vi "PS-OCTA-OCE-autofocus.vi"() -> ()   [LabVIEW 2024] (continued)
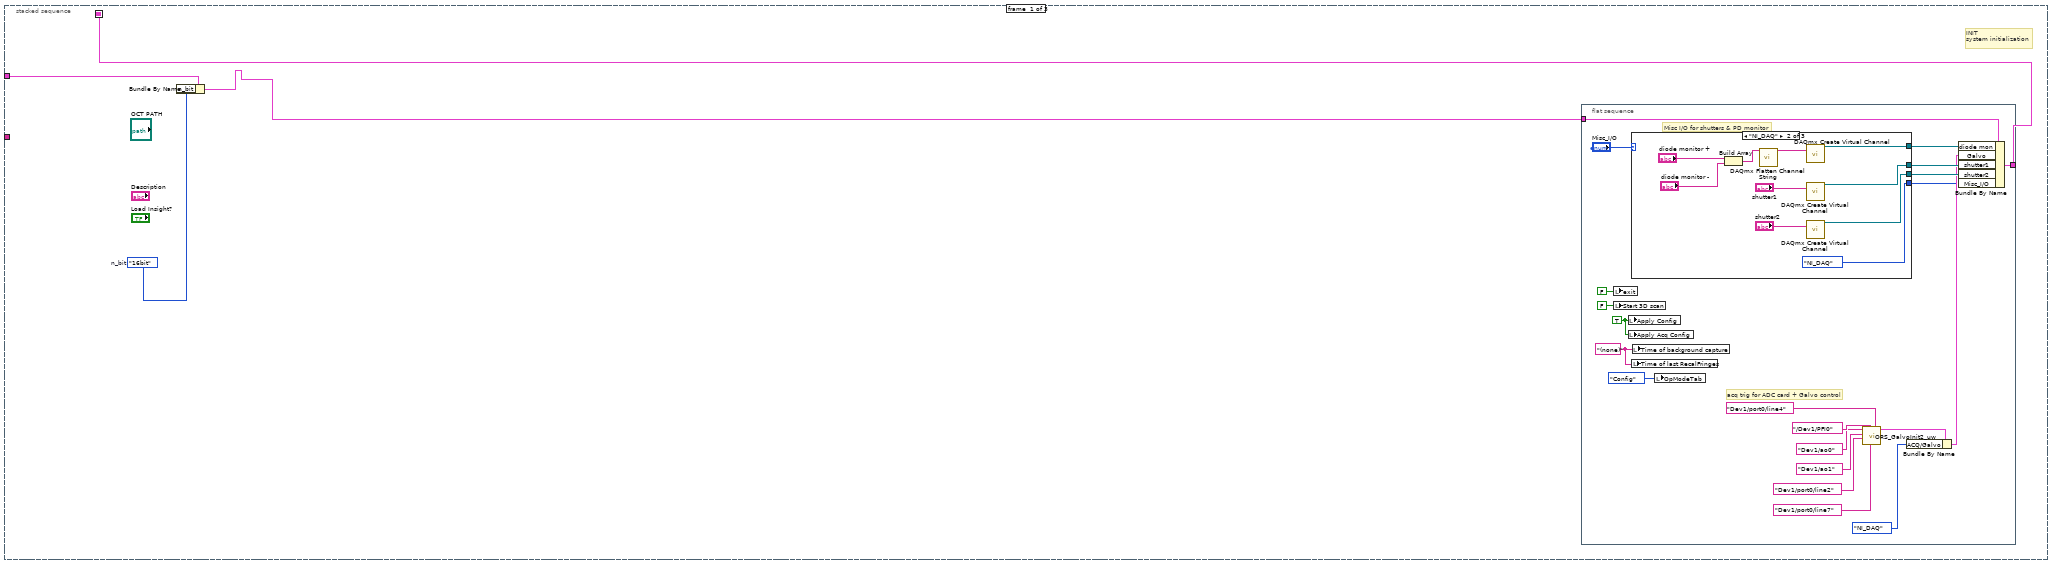
[diagram p3: hidden frame]
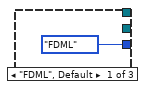
[diagram p4: hidden frame]
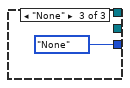
[diagram p5: hidden frame]
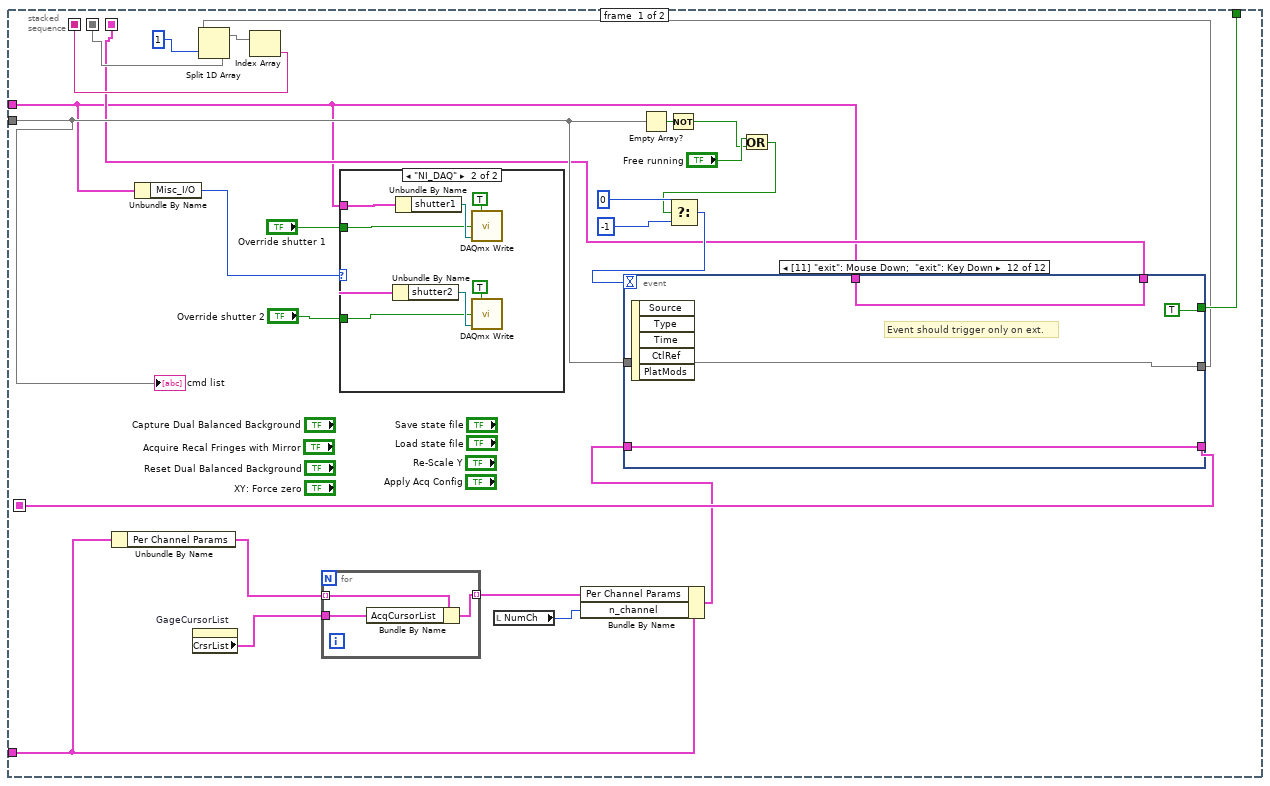
[diagram p7: hidden frame]
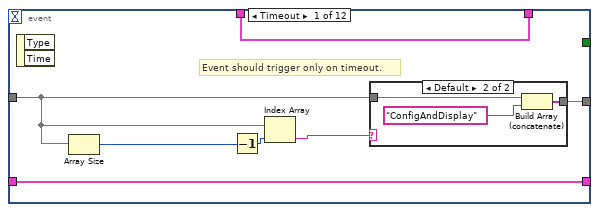
[diagram p9: hidden frame]
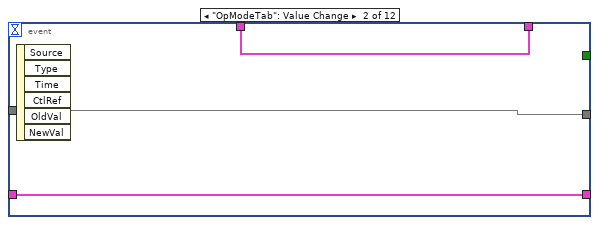
[diagram p11: hidden frame]
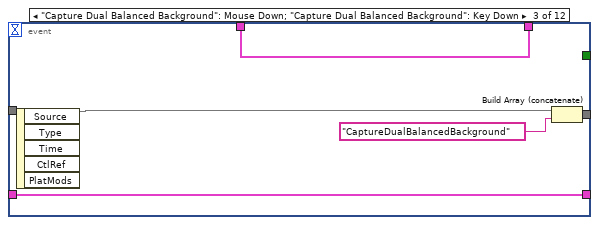
[diagram p12: hidden frame]
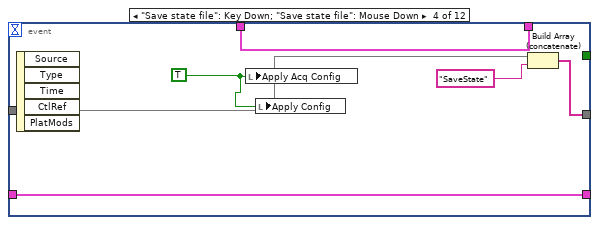
[diagram p13: hidden frame]
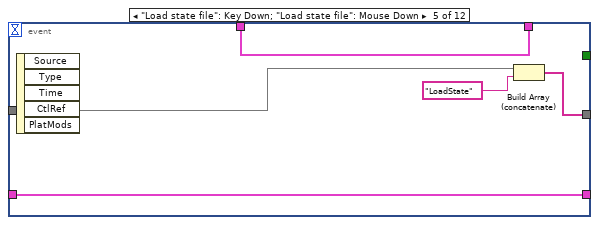
[diagram p14: hidden frame]
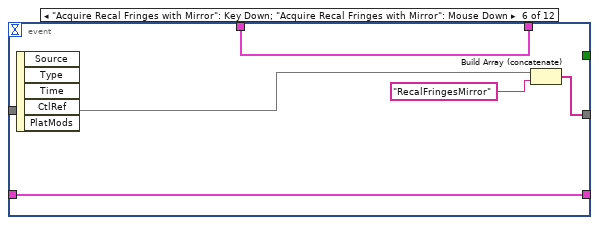
[diagram p15: hidden frame]
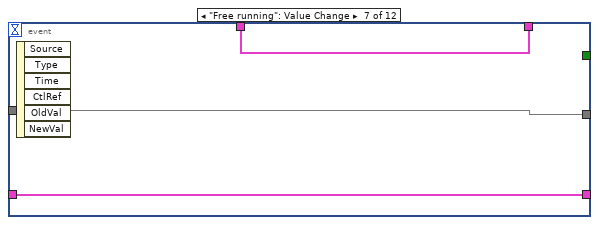
[diagram p16: hidden frame]
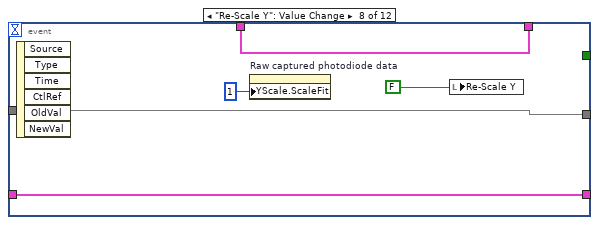
[diagram p17: hidden frame]
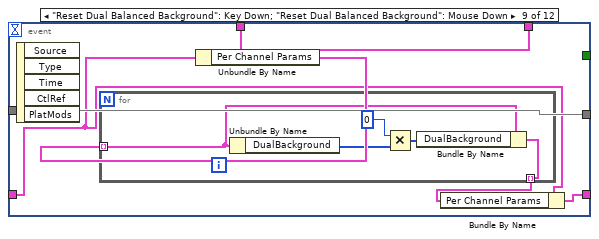
[diagram p18: hidden frame]
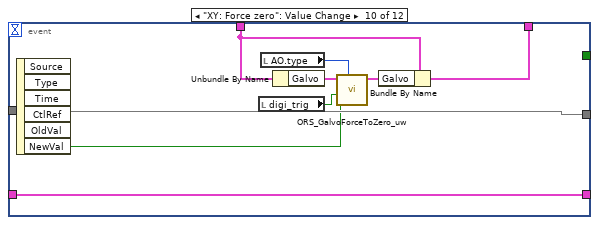
[diagram p19: hidden frame]
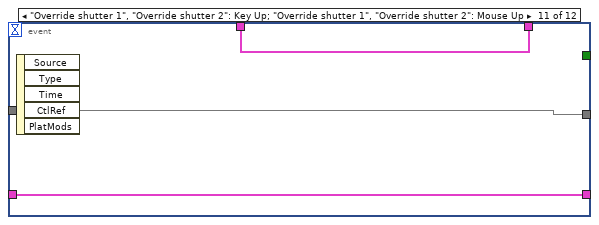
[diagram p20: hidden frame]
                    # "data transfer end timer"
                    # "acq start timer"
                    # "#AllocatedBuffer"
                    n725 = stacked-sequence {
                      seq-local: [_ w1514 _ _ _] -> [_ _ w1706 _ _]
                      seq-local: [_ w1520 _ _ _] -> [_ _ w1703 _ w1985]
                      seq-local: [_ w1519 _ _ _] -> [_ _ w1702 _ _]
                      seq-local: [_ w1518 _ _ _] -> [_ _ _ w1961 _]
                      seq-local: [_ _ w1701 _ _] -> [_ _ _ w1960 _]
                      seq-local: [_ _ w1700 _ _] -> [_ _ _ w1955 _]
                      seq-local: [_ _ w1699 _ _] -> [_ _ _ w1953 _]
                      seq-local: [_ _ w1698 _ _] -> [_ _ _ w1957 _]
                      seq-local: [_ w1517 _ _ _] -> [_ _ w1697 _ _]
                      seq-local: [_ w1516 _ _ _] -> [_ _ _ w1950 _]
                      seq-local: [_ w1515 _ _ _] -> [_ _ w1691 _ _]
                      seq-local: [_ w1513 _ _ _] -> [_ _ w1696 _ _]
                      seq-local: [_ w1512 _ _ _] -> [_ _ w1695 _ _]
                      seq-local: [_ w1511 _ _ _] -> [_ _ w1694 _ _]
                      seq-local: [_ w1510 _ _ _] -> [_ _ w1693 _ _]
                      seq-local: [_ w1509 _ _ _] -> [_ _ w1692 _ _]
                      seq-local: [w1499 _ _ _ _] -> [_ w1508 _ _ _]
                      seq-local: [_ w1507 _ _ _] -> [_ _ w1690 _ _]
                      tunnel: w1496 -> [w1502 _ _ _ _]
                      tunnel: [_ _ _ _ w1987] -> w1495
                      tunnel: w1494 -> [_ w1521 w1707 _ w1975]
                      tunnel: [_ _ _ _ w1975] -> w1493
                      tunnel: w1492 -> [_ _ w1705 _ _]
                      tunnel: w1491 -> [_ _ w1704 _ _]
                      frame #0 {
                        n726 = local read "ATSHandle"() -> (w1497:u32[])
                        n727 = Unbundle By Name(w1502) -> ("Galvo"=w1500:T5)
                        n728 = call "ORS_GalvoCleanupScan.vi"("Galvo"=w1500) -> ("Galvo out"=w1501:T5)  [unwired: 9 in, 1 out]
                        n729 = for {
                          tunnel: [w1506] -> w1498
                          tunnel: w1497 -> [w1503] mode=indexing
                          n730 = call "AlazarAbortCapture.vi"("Handle"=w1503) -> ("Handle"=w1505:u32, "error out"=w1504:errorcluster)  [unwired: 1 in, 1 out]
                          n731 = call "AlazarAbortAsyncRead.vi"("Handle"=w1505, "error in (no error)"=w1504) -> ("error out"=w1506:errorcluster)  [unwired: 2 out]
                        }
                        n732 = Bundle By Name(cluster=w1502, "Galvo"=w1501) -> (w1499:T6)
                        n733 = call <vilib>:"Simple Error Handler.vi"("error in (no error)"=w1498) -> ()  [unwired: 4 in, 5 out]
                      }
                      frame #1 {
                        n734 = stacked-sequence {
                          seq-local: [w1556 _ _ _ _] -> [_ w1625 _ _ _]
                          seq-local: [w1548 _ _ _ _] -> [_ w1629 _ _ _]
                          seq-local: [w1547 _ _ _ _] -> [_ w1628 _ _ _]
                          seq-local: [w1546 _ _ _ _] -> [_ w1627 _ _ _]
                          seq-local: [w1542 _ _ _ _] -> [_ w1626 _ _ _]
                          seq-local: [w1541 _ _ _ _] -> [_ w1588 _ _ _]
                          seq-local: ["3D frame" _ _ _ _] -> [_ w1608 _ _ _]
                          seq-local: ["B_frames per trigger" _ _ _ _] -> [_ w1607 _ _ _]
                          seq-local: [_ w1629 _ _ _] -> [_ _ w1676 _ _]
                          seq-local: [_ w1625 _ _ _] -> [_ _ w1675 _ _]
                          seq-local: [_ w1628 _ _ _] -> [_ _ w1674 _ _]
                          seq-local: [_ w1627 _ _ _] -> [_ _ w1673 _ _]
                          seq-local: [_ _ w1675 _ _] -> [_ _ _ w1684 _]
                          seq-local: [_ _ _ w1684 _] -> [_ _ _ _ w1687]
                          tunnel: w1508 -> [w1557 _ _ _ _]
                          tunnel: w1521 -> [w1541 _ _ _ _]
                          tunnel: [w1548 _ _ _ _] -> w1519
                          tunnel: [w1545 _ _ _ _] -> w1517
                          tunnel: [w1535 _ _ _ _] -> w1515
                          tunnel: [w1543 _ _ _ _] -> w1514
                          tunnel: [w1539 _ _ _ _] -> w1507
                          tunnel: [_ w1610 _ _ _] -> w1513
                          tunnel: [_ w1612 _ _ _] -> w1512
                          tunnel: [_ w1624 _ _ _] -> w1511
                          tunnel: [_ w1623 _ _ _] -> w1510
                          tunnel: [_ w1616 _ _ _] -> w1509
                          tunnel: [_ _ w1672 _ _] -> w1516
                          tunnel: [_ _ _ _ w1686] -> w1520
                          tunnel: [_ _ _ _ w1685] -> w1518
                          frame #0 {
                            (unwired) u32 0 ("y")
                            w1538 = 10178 items=["Finite Samples"=10178, "Continuous Samples"=10123, "Hardware Timed Single Point"=12522] ("SampQuant.SampMode")
                            # "Trigger condition: 0 =  transducer ON for the scan"
                            n735 = case shown="False" "3D: dummy/real" {
                              tunnel: [w1560 w1561] -> w1548
                              tunnel: T12."Alazar" ("Data source") -> [w1558 w1561]
                              frame False {
                                n736 = Type Cast(type=w1558, x=9999) -> (*(type *) &x=w1560:T12)
                              }
                              frame True {
                              }
                            }
                            n737 = Unbundle By Name(w1557) -> ("Galvo"=w1552:T5)
                            n738 = local read "3D_Galvo_Params"() -> (w1527:T4)
                            n739 = local read "XY: Force zero"() -> (w1551:bool)
                            n740 = Bundle By Name(cluster=w1552, "params"=w1527, "params.force to zero"=w1551, "params.Triggers_per_sweep"=1.0) -> (w1550:T5)
                            n741 = Unbundle By Name(w1527) -> ("mode"=w1525:i32)
                            n742 = Subtract(x=w1525, y=7) -> (x-y=w1523:i32)
                            n743 = Multiply(x=w1523, y=-1) -> (x*y=w1522:i32)
                            n744 = local read "digi_trig"() -> (w1537:bool)
                            n745 = call "ORS_GalvoConfig3D_v2.vi"("Galvo"=w1550, "use_digi_trig"=w1537) -> ("Galvo out"=w1531:T5, "error out"=w1554:errorcluster)  [unwired: 16 in]
                            n746 = local read "Slow axis-----Fast axis"() -> (w1528:bool)
                            n747 = local read "AO.type"() -> (w1533:i32)
                            n748 = call "ORS_GalvoPrepareScan_uw-1kp_Duo.vi"("Galvo"=w1531, "SampQuant.SampMode"=w1538, "3D frame"="3D frame", "AO.DataXferMech"=w1533, "Fast Axis/Slow Axis"=w1528, "use_digi_trig"=w1537, "error in"=w1554, "Trigger condition"=w1522) -> ("Galvo out"=w1532:T5, "error out"=→"error out":errorcluster)  [unwired: 4 in, 2 out]
                            n749 = Unbundle By Name(w1532) -> ("params.n_lines"=w1553:i32, "params.n_frames"=w1536:i32)
                            n750 = Bundle By Name(cluster=w1557, "Galvo"=w1532) -> (w1556:T6)
                            n751 = case shown="\"Alazar\"" w1548 {
                              tunnel: w1536 -> [_ w1576]
                              tunnel: w1553 -> [_ w1579]
                              tunnel: [-1.0 w1573] -> w1542
                              tunnel: [_ w1565] -> w1547
                              tunnel: [_ w1578] -> w1546
                              tunnel: [_ w1575] -> w1545
                              tunnel: [_ w1574] -> w1543
                              tunnel: [_ w1567] -> w1539
                              tunnel: [_ w1566] -> w1534
                              frame Default {
                              }
                              frame "Alazar" {
                                n752 = Multiply(x=w1576, y=w1579) -> (x*y=w1571:i32)
                                n753 = Multiply(x=w1571, y=1) -> (x*y=w1570:i32)
                                n754 = local read "Laser Trigger"() -> (w1563:bool)
                                n755 = local read "ATSHandle"() -> (w1565:u32[])
                                n756 = local read "# samples"() -> (w1573:u32)
                                n757 = local read "Channel"() -> (w1572:u32)
                                n758 = for {
                                tunnel: w1565 -> [w1587] mode=indexing
                                tunnel: w1579 -> [w1586]
                                tunnel: [w1585] -> w1578
                                tunnel: w1573 -> [w1584]
                                tunnel: w1572 -> [w1583]
                                tunnel: w1570 -> [w1582]
                                tunnel: [w1581] -> w1564
                                tunnel: w1563 -> [w1580]
                                n759 = call "ORS_AlazarDLLAcq_Prepare.vi"("Lamda Trigger?"=w1580, "Channel"=w1583, "Records Per Buffer"=w1586, "Records Count"=w1582, "Record length"=w1584, "ATSHandle"=w1587) -> ("error out"=w1585:errorcluster, "Samps Per Buffer"=w1581:u32)  [unwired: 3 in, 1 out]
                                }
                                n760 = Array Size(array=w1565) -> (size(s)=w1566:i32)
                                n761 = Multiply(x=w1564, y=w1566) -> ()  [unwired: 1 out]
                                n762 = Initialize Array(i16 0 ("element"), w1564) -> (w1575:i16[])
                                n763 = Obtain Queue(element data type=w1575) -> (queue out=w1574:refnum<queue>)  [unwired: 4 in, 2 out]
                                n764 = Multiply(x=w1564, y=u32 2) -> (x*y=w1567:u32)
                              }
                            }
                            "samples/line 3d" <- w1542
                            n765 = Multiply(x=w1536, y=w1534) -> (x*y=w1535:i32)
                          }
                          frame #1 {
                            # "File suffix to add angle, type of acquisition and extension to the file name"
                            n766 = local read "OCTA_indicator"() -> (w1595:bool)
                            n767 = local read "Current Angle"() -> (w1605:dbl)
                            n768 = call "ORS_timestamp.vi"() -> ("system time"=w1620:string)
                            n769 = call "ORS_DatafileWriteReadHeader_OCE.vi"() -> ("Parameter Cluster v8"=w1609:T27, "error out"=w1606:errorcluster)  [unwired: 17 in, 1 out]
                            n770 = stacked-sequence {
                              seq-local: [w1640 _] -> [_ w1650]
                              tunnel: w1609 -> [w1634 _]
                              tunnel: w1625 -> [w1642 _]
                              tunnel: w1626 -> [w1641 _]
                              tunnel: [_ w1653] -> w1613
                              tunnel: w1588 -> [w1638 w1652]
                              tunnel: [_ w1647] -> w1623
                              tunnel: [_ w1645] -> w1624
                              tunnel: [_ w1644] -> w1616
                              frame #0 {
                                n771 = Unbundle By Name(w1638) -> ("Sample Rate"=w1639:dbl)
                                n772 = local read "Description"() -> (w1630:string)
                                n773 = local read "file version"() -> (w1636:u32)
                                n774 = local read "image height"() -> (w1635:i32)
                                n775 = Unbundle By Name(w1642) -> ("Galvo"=w1633:T5)
                                n776 = local read "n_bit"() -> (w1632:enum16{"8bit", "16bit"})
                                n777 = Bundle By Name(cluster=w1634, "Galvo"=w1633, "description"=w1630, "samples_per_line"=w1641, "sampling_rate"=w1639, "vert_range"=0.0, "image height (crop)"=w1635, "file version"=w1636, "data set dimension"=u16 1, "n_bit"=w1632) -> (w1640:T27)
                              }
                              frame #1 {
                                n778 = Unbundle By Name(w1652) -> ("Per Channel Params"=w1649:T8)
                                n779 = Index Array(array=w1649) -> (element=w1643:T13)  [unwired: 1 in]
                                n780 = local read "DoInterp"() -> (w1646:bool)
                                n781 = local read "NumCh"() -> (w1651:i32)
                                n782 = Unbundle By Name(w1643) -> ("DualBackground"=w1644:i16[], "RecalFringePhaseFit"=w1648:dbl[][])
                                n783 = Bundle By Name(cluster=w1650, "n_channel"=w1651, "Per Channel Params"=w1649) -> (w1653:T27)
                                n784 = case shown="False" w1646 {
                                tunnel: w1648 -> [w1656 w1665]
                                tunnel: [w1655 w1663] -> w1647
                                tunnel: [w1654 w1663] -> w1645
                                frame True {
                                n785 = Index Array(array=w1656, index (row)=0) -> (element=w1654:dbl[])  [unwired: 1 in]
                                n786 = Array Size(array=w1654) -> (size(s)=w1660:i32)
                                n787 = Decrement(x=w1660) -> (x-1=w1662:i32)
                                n788 = Index Array(array=w1654, index #1=0 ("index"), index #2=w1662) -> (element #1=w1658:dbl, element #2=w1659:dbl)
                                n789 = call-poly <vilib>:"Ramp Pattern.vi"("start"=w1658, "end"=w1659, "samples"=w1660) -> ("Ramp Pattern"=w1655:dbl[])  [unwired: 7 in, 1 out]
                                }
                                frame False {
                                n790 = Index Array(array=w1665, index (row)=0) -> (element=w1664:dbl[])  [unwired: 1 in]
                                n791 = Array Size(array=w1664) -> (size(s)=w1669:i32)
                                n792 = Decrement(x=w1669) -> (x-1=w1671:i32)
                                n793 = Index Array(array=w1664, index #1=0 ("index"), index #2=w1671) -> (element #1=w1667:dbl, element #2=w1668:dbl)
                                n794 = call-poly <vilib>:"Ramp Pattern.vi"("start"=w1667, "end"=w1668, "samples"=w1669) -> ("Ramp Pattern"=w1663:dbl[])  [unwired: 7 in, 1 out]
                                }
                                }
                              }
                            }
                            n795 = Append True/False String(1:w1595, 2:" ", 3:"_OCTA_") -> (0:w1597:string)  [unwired: 1 in]
                            n796 = Select(t=w1620, s="timestamp? 3d", f="") -> (s? t:f=w1621:string)
                            n797 = local read "OCE_indicator"() -> (w1589:bool)
                            n798 = Append True/False String(1:w1589, 2:" ", 3:"_OCE_", 4:w1597) -> (0:w1596:string)
                            n799 = local read "OCT indicator"() -> (w1594:bool)
                            n800 = Append True/False String(1:w1594, 2:" ", 3:"_OCT_", 4:w1596) -> (0:w1593:string)
                            n801 = Number To Decimal String(number=w1605, width (-)=i16 3) -> (decimal integer string=w1592:string)
                            n802 = Concatenate Strings(w1593, w1592, ".oct" ("string")) -> (w1590:string)
                            "OCT FILE extension" <- w1590
                            n803 = Concatenate Strings(w1621, "OCT NAME", w1590) -> (w1622:string)
                            n804 = local read "OCT PATH"() -> (w1615:path)
                            n805 = Build Path(base path=w1615, name or relative path=w1622) -> (appended path=w1614:path)
                            n806 = call "ORS_DatafileWriteReadHeader_OCE.vi"("file path"=w1614, "3D frame"=w1608, "read/write"="data ver", "B_frame_per_trigger"=w1607, "error in"=w1606, "Parameter Cluster v8"=w1613) -> ("file refnum"=w1610:refnum<file>, "error out"=w1612:errorcluster)  [unwired: 11 in, 1 out]
                          }
                          frame #2 {
                            n807 = case shown="\"Alazar\"" w1676 {
                              tunnel: w1674 -> [_ w1679]
                              tunnel: w1673 -> [_ w1678]
                              tunnel: [_ w1677] -> w1672
                              frame Default {
                              }
                              frame "Alazar" {
                                n808 = for {
                                tunnel: w1679 -> [w1682] mode=indexing
                                shift-right: [w1680] -> w1677
                                shift-left: w1678 -> [w1681]
                                n809 = call "ORS_AlazarDLLAcq_Start.vi"("error in (no error)"=w1681, "ATSHandle"=w1682) -> ("error out"=w1680:errorcluster)  [unwired: 8 in, 1 out]
                                }
                              }
                            }
                          }
                          frame #3 {
                            n810 = Wait (ms)(milliseconds to wait=u32 1000) -> ()  [unwired: 1 out]
                          }
                          frame #4 {
                            n811 = Unbundle By Name(w1687) -> ("Galvo"=w1689:T5)
                            n812 = call "ORS_GalvoStartScan.vi"("Galvo"=w1689) -> ("Galvo out"=w1688:T5)  [unwired: 9 in, 1 out]
                            n813 = Bundle By Name(cluster=w1687, "Galvo"=w1688) -> (w1686:T6)
                            n814 = Tick Count (ms)() -> (millisecond timer value=w1685:u32)
                          }
                        }
                      }
                      frame #2 {
                        n815 = stacked-sequence {
                          seq-local: [w1724 _ _] -> [_ w1801 _]
                          seq-local: [w1723 _ _] -> [_ w1800 _]
                          seq-local: [w1719 _ _] -> [_ w1795 _]
                          seq-local: [dbl[][] [] _ _] -> [_ w1799 _]
                          seq-local: [w1721 _ _] -> [_ w1798 _]
                          seq-local: [w1718 _ _] -> [_ w1794 _]
                          seq-local: [w1717 _ _] -> [_ w1793 _]
                          seq-local: [w1716 _ _] -> [_ w1792 _]
                          seq-local: [w1710 _ _] -> [_ w1791 _]
                          seq-local: [_ w1797 _] -> [_ _ w1949]
                          seq-local: [_ w1796 _] -> [_ _ w1948]
                          seq-local: [_ w1789 _] -> [_ _ w1947]
                          tunnel: w1707 -> [_ _ _]
                          tunnel: w1706 -> [w1715 _ _]
                          tunnel: w1705 -> [_ _ _]
                          tunnel: w1704 -> [_ _ _]
                          tunnel: w1703 -> [w1725 _ _]
                          tunnel: w1702 -> [w1713 _ _]
                          tunnel: [w1720 _ _] -> w1701
                          tunnel: w1697 -> [w1714 _ _]
                          tunnel: w1691 -> [w1709 _ _]
                          tunnel: w1690 -> [w1708 _ _]
                          tunnel: w1703 -> [_ w1802 _]
                          tunnel: w1691 -> [_ w1790 _]
                          tunnel: w1696 -> [_ w1786 _]
                          tunnel: w1695 -> [_ w1785 _]
                          tunnel: w1694 -> [_ w1784 _]
                          tunnel: w1693 -> [_ w1783 _]
                          tunnel: w1692 -> [_ w1782 _]
                          tunnel: [_ _ w1949] -> w1700
                          tunnel: [_ _ w1948] -> w1699
                          frame #0 {
                            n816 = flat-sequence {
                              tunnel: w1725 -> [w1734]
                              tunnel: w1715 -> [w1733]
                              tunnel: w1714 -> [w1732]
                              tunnel: w1713 -> [w1731]
                              tunnel: [w1730] -> w1711
                              tunnel: w1709 -> [w1729]
                              tunnel: w1708 -> [w1728]
                              tunnel: [w1777] -> w1720
                              tunnel: [w1776] -> w1712
                              tunnel: w1711 -> [w1776]
                              tunnel: [w1778] -> w1710
                              tunnel: w1712 -> [w1778]
                              frame #0 {
                                n817 = case shown="\"Alazar\"" w1731 {
                                tunnel: w1733 -> [_ w1740]
                                tunnel: w1734 -> [w1735 _]
                                tunnel: w1732 -> [_ w1739]
                                tunnel: [_ w1741] -> w1730
                                tunnel: w1729 -> [_ w1736]
                                tunnel: w1728 -> [_ w1738]
                                frame Default {
                                # "FIXME: We should simply wait for the DAQ taks to finish!"
                                n818 = Unbundle By Name(w1735) -> ()  [unwired: 3 out]
                                }
                                frame "Alazar" {
                                n819 = local read "ATSHandle"() -> (w1737:u32[])
                                n820 = while {
                                shift-right: [w1749] -> w1741
                                shift-left: w1740 -> [w1751]
                                shift-right: [w1747] -> _
                                shift-left: u32 0 ("new element/subarray") -> [w1750]
                                tunnel: w1739 -> [w1748]
                                tunnel: w1736 -> [w1746]
                                tunnel: w1738 -> [w1744]
                                tunnel: w1737 -> [w1743]
                                stop <- w1745 stop-if-true
                                n821 = for {
                                tunnel: w1748 -> [w1762]
                                tunnel: w1746 -> [w1755]
                                tunnel: [w1760] -> w1745
                                tunnel: w1744 -> [w1758]
                                tunnel: w1743 -> [w1756] mode=indexing
                                shift-right: [w1763] -> w1749
                                shift-left: w1751 -> [w1765]
                                shift-right: [w1761] -> w1747
                                shift-left: w1750 -> [w1764]
                                n822 = call "AlazarWaitNextAsyncBufferCompleteI16.vi"("bytesToCopy"=w1758, "timeout_ms"=u32 0, "Buffer"=w1762, "Handle"=w1756) -> ("Return Code"=w1759:u32, "Buffer"=w1753:u16[])  [unwired: 1 in, 1 out]
                                n823 = Subtract(x=w1753, y=32768.0) -> (x-y=w1752:i16[])
                                n824 = case shown="512, 589" w1759 {
                                selector: w1759 -> [w1766 _]
                                tunnel: w1752 -> [_ w1772]
                                tunnel: w1765 -> [w1767 w1773]
                                tunnel: w1764 -> [w1768 w1775]
                                tunnel: [w1768 w1771] -> w1761
                                tunnel: [w1767 w1774] -> w1763
                                tunnel: w1759 -> [_ _]
                                tunnel: w1755 -> [_ w1769]
                                frame 0, Default {
                                "Return Code" <- w1766
                                }
                                frame 512, 589 {
                                n825 = Enqueue Element(queue=w1773, element=w1772) -> (queue out=w1774:refnum<queue>)  [unwired: 2 in, 2 out]
                                n826 = Increment(x=w1775) -> (x+1=w1771:u32)
                                n827 = Divide(x=w1771, y=w1769) -> (x/y=→"#Done":dbl)
                                }
                                }
                                n828 = Equal?(x=w1761, y=w1755) -> (x = y?=w1760:bool)
                                }
                                }
                                }
                                }
                              }
                              frame #1 {
                                n829 = Tick Count (ms)() -> (millisecond timer value=w1777:u32)
                              }
                              frame #2 {
                                n830 = call <vilib>:"Beep.vi"("use system alert? (T)"=FALSE, "duration (msec)"=u32 100, "frequency (Hz)"=u32 2000) -> ()  [unwired: 9 in]
                              }
                            }
                            n831 = Unbundle By Name(w1725) -> ("Galvo.params.n_lines"=w1719:i32)
                            n832 = property on="Raw captured photodiode data" class="WFGraph (strict)"() -> ("CrsrList"=w1727:T9)  [unwired: 2 in, 2 out]
                            n833 = local read "crop start"() -> (w1723:i32)
                            n834 = local read "samples/line 3d"() -> (w1718:dbl)
                            n835 = local read "image height"() -> (w1724:i32)
                            n836 = call "ORS_CursorToCropIdx.vi"("index offset"=0, "Cursor List"=w1727) -> ("length"=w1716:i32, "offset"=w1717:i32)  [unwired: 8 in]
                            n837 = Tick Count (ms)() -> (millisecond timer value=w1721:u32)
                          }
                          frame #1 {
                            n838 = for {
                              N: w1790 -> [w1814]
                              shift-right: [w1845] -> w1797
                              shift-left: w1786 -> [w1847]
                              shift-right: [w1844] -> w1796
                              shift-left: w1785 -> [w1846]
                              shift-right: [w1841] -> _
                              shift-left: w1798 -> [w1842]
                              tunnel: w1801 -> [w1840]
                              tunnel: w1800 -> [w1839]
                              tunnel: w1795 -> [w1838]
                              shift-right: [w1837] -> _
                              shift-left: w1799 -> [w1836]
                              tunnel: w1802 -> [w1825]
                              tunnel: w1793 -> [w1819]
                              tunnel: w1792 -> [w1818]
                              tunnel: w1794 -> [w1817]
                              tunnel: w1783 -> [w1816]
                              tunnel: w1784 -> [w1815]
                              tunnel: w1791 -> [w1812]
                              tunnel: [w1810] -> w1789
                              tunnel: w1782 -> [w1809]
                              i -> [w1813]
                              stop <- "cancel 3D" stop-if-true
                              w1821 = 50 ("y")
                              # "Process and write frame after frame"
                              # "write frames"
                              n839 = local read "3D_Galvo_Params"() -> (w1808:T4)
                              n840 = Dequeue Element(queue=w1812) -> (queue out=w1810:refnum<queue>, element=w1811:i16[])  [unwired: 2 in, 2 out]
                              n841 = Unbundle By Name(w1825) -> ("n_bit"=w1822:enum16{"8bit", "16bit"})
                              "n_bit" <- w1822
                              n842 = Select(t=1.0, s="even/odd", f=0.0) -> (s? t:f=w1829:dbl)
                              n843 = Increment(x=w1813) -> (x+1=w1824:i32)
                              n844 = Add(x=w1829, y=w1824) -> (x+y=w1827:dbl)
                              n845 = Quotient & Remainder(x=w1824, y=w1821) -> (x-y*floor(x/y)=w1823:i32)  [unwired: 1 out]
                              n846 = Wait (ms)(milliseconds to wait="preview delay (ms)") -> ()  [unwired: 1 out]
                              n847 = Unbundle By Name(w1808) -> ("f_per_pos"=w1807:i32)
                              n848 = Array Size(array=w1811) -> (size(s)=w1820:i32)
                              n849 = Quotient & Remainder(x=w1827, y=w1807) -> (x-y*floor(x/y)=w1826:dbl)  [unwired: 1 out]
                              n850 = case shown="True" "Write data?" {
                                tunnel: w1847 -> [w1867 w1873]
                                tunnel: w1846 -> [w1866 w1872]
                                tunnel: [w1867 w1871] -> w1845
                                tunnel: [w1866 w1870] -> w1844
                                tunnel: w1822 -> [_ _]
                                tunnel: w1811 -> [_ w1869]
                                frame False {
                                }
                                frame True {
                                n851 = local read "data ver"() -> (w1868:u16)
                                n852 = call "ORS_DatafileWriteData-v2.vi"("data ver"=w1868, "error in"=w1872, "frame data"=w1869, "file refnum"=w1873) -> ("error out"=w1870:errorcluster, "file refnum"=w1871:refnum<file>)  [unwired: 6 in]
                                }
                              }
                              n853 = case shown="0" w1823 {
                                tunnel: w1842 -> [w1849 w1864]
                                tunnel: [w1849 w1863] -> w1841
                                tunnel: w1820 -> [_ w1858]
                                tunnel: w1814 -> [_ w1857]
                                tunnel: w1824 -> [_ w1856]
                                tunnel: w1822 -> [_ w1852]
                                tunnel: w1821 -> [_ w1853]
                                frame Default {
                                }
                                frame 0 {
                                n854 = Divide(x=w1856, y=w1857) -> (x/y=→"Progress":dbl)
                                n855 = To Long Integer(number=w1852) -> (32bit integer=w1851:i32)
                                n856 = Divide(x=1024.0 ("y"), y=w1853) -> (x/y=w1854:dbl)
                                n857 = Increment(x=w1851) -> (x+1=w1850:i32)
                                n858 = Tick Count (ms)() -> (millisecond timer value=w1863:u32)
                                n859 = Subtract(x=w1863, y=w1864) -> (x-y=w1862:u32)
                                n860 = Multiply(x=w1858, y=w1850) -> (x*y=w1861:i32)
                                n861 = Divide(x=w1861, y=w1862) -> (x/y=w1860:dbl)
                                n862 = Divide(x=w1860, y=w1854) -> (x/y=→"data rate":dbl)
                                "frame size 3d" <- w1858
                                }
                              }
                              n863 = Equal To 0?(x=w1826) -> (x = 0?=w1834:bool)
                              n864 = And(x="Display 3d data", y=w1834) -> (x .and. y?=w1832:bool)
                              n865 = case shown="True" w1832 {
                                tunnel: w1811 -> [_ w1897]
                                tunnel: w1840 -> [_ w1886]
                                tunnel: w1839 -> [_ w1910]
                                tunnel: w1838 -> [_ w1887]
                                tunnel: [w1874 w1909] -> w1837
                                tunnel: w1836 -> [w1874 w1906]
                                tunnel: w1819 -> [_ w1895]
                                tunnel: w1818 -> [_ w1894]
                                tunnel: w1817 -> [_ w1896]
                                tunnel: w1816 -> [_ w1878]
                                tunnel: w1815 -> [_ w1879]
                                tunnel: w1809 -> [_ w1877]
                                frame False {
                                }
                                frame True {
                                # "update every 4th"
                                n866 = Array Size(array=w1906) -> (size(s)=w1905:i32[])
                                n867 = local read "Enable DVV?"() -> (w1880:bool)
                                n868 = local read "cut_level_high"() -> (w1885:dbl)
                                n869 = local read "cut_level_low"() -> (w1884:dbl)
                                n870 = case shown="True" w1880 {
                                tunnel: w1897 -> [w1911 w1912]
                                tunnel: [w1911 w1916] -> w1898
                                tunnel: w1895 -> [_ w1914]
                                tunnel: w1894 -> [_ w1915]
                                tunnel: w1887 -> [_ w1913]
                                frame False {
                                }
                                frame True {
                                n871 = local read "Data Valid Vector"() -> (w1917:u32[])
                                n872 = local read "samples/line 3d"() -> (w1919:dbl)
                                n873 = local read "DVV shift"() -> (w1918:i32)
                                n874 = call "ORS_Insight_Reduce_B-scan_Data.vi"("length"=w1915, "offset"=w1914, "Data Valid Vector"=w1917, "spl per line"=w1919, "DVV shift"=w1918, "line Num"=w1913, "Input"=w1912) -> ("Output"=w1916:i16[])  [unwired: 4 in]
                                }
                                }
                                n875 = Bundle("samples/line 3d"=w1896, "n_lines"=w1887, "cut_level_high"=w1885, "cut_level_low"=w1884, "offset"=w1895, "length"=w1894, "crop start"=w1910, "image height"=w1886) -> (w1883:T28)  [unwired: 1 in]
                                n876 = local read "PhaseCompVector"() -> (w1875:cdb[])
                                n877 = local read "FFT Down Sample"() -> (w1881:i32)
                                n878 = local read "DoDispComp"() -> (w1876:bool)
                                n879 = local read "DoInterp"() -> (w1882:bool)
                                n880 = call "ORS_UW_ImgGen.vi"("Disp Comp"=w1876, "Phase Comp Vector"=w1875, "xi"=w1878, "Do Interp"=w1882, "X"=w1879, "imgGen Control"=w1883, "FFT Down Sample"=w1881, "DualBackground"=w1877, "Raw Input"=w1898) -> ("output array"=w1889:u8[])  [unwired: 1 in, 1 out]
                                n881 = Index Array(array=w1905) -> (element #1=w1900:i32, element #2=w1901:i32)  [unwired: 2 in]
                                n882 = Reshape Array(w1889, w1887, w1886) -> (w1890:u8[][])
                                n883 = Multiply(x=w1900, y=w1901) -> (x*y=w1904:i32)
                                n884 = Transpose 2D Array(2D array=w1890) -> (transposed array=w1893:u8[][])
                                n885 = Array Size(array=w1890) -> (size(s)=w1891:i32[])
                                n886 = Multiply Array Elements(1:w1891) -> (0:w1892:i32)
                                n887 = And(x=w1900, y=3) -> (x .and. y?=w1902:i32)
                                n888 = local read "cmap"() -> (w1908:string)
                                n889 = Reshape Array(w1893, w1892) -> (w1888:u8[])
                                n890 = call "ORS_DrawFlattenedPixmap8.vi"("colormap data string"=w1908, "height"=w1886, "width"=w1887, "image data"=w1888) -> ("new picture"=w1899:picture)  [unwired: 5 in]
                                n891 = case shown="True" "en face?" {
                                tunnel: w1888 -> [_ w1933]
                                tunnel: w1886 -> [_ w1932]
                                tunnel: w1887 -> [_ w1927]
                                tunnel: [w1920 w1929] -> w1909
                                tunnel: w1906 -> [w1920 w1930]
                                tunnel: w1908 -> [_ w1928]
                                tunnel: w1901 -> [_ w1926]
                                tunnel: w1904 -> [_ w1925]
                                tunnel: w1900 -> [_ w1924]
                                tunnel: w1902 -> [_ w1923]
                                frame False {
                                }
                                frame True {
                                n892 = Reshape Array(w1933, w1932, w1927) -> (w1922:u8[][])
                                n893 = Transpose 2D Array(2D array=w1922) -> (transposed array=w1921:u8[][])
                                n894 = for {
                                tunnel: w1921 -> [w1946] mode=indexing
                                tunnel: [w1945] -> w1931 mode=indexing
                                n895 = call-poly <vilib>:"Mean.vi"("X"=w1946) -> ("mean"=w1945:dbl)  [unwired: 1 out]
                                }
                                n896 = Build Array (concatenate)(w1930, w1931) -> (w1929:dbl[][])
                                n897 = case shown="0" w1923 {
                                tunnel: w1929 -> [_ w1940]
                                tunnel: w1928 -> [_ w1944]
                                tunnel: w1926 -> [_ w1941]
                                tunnel: w1925 -> [_ w1943]
                                tunnel: w1924 -> [_ w1942]
                                frame Default {
                                }
                                frame 0 {
                                n898 = Reshape Array(w1940, w1943) -> (w1936:dbl[])
                                n899 = Array Max & Min(array=w1940) -> (max value=w1939:dbl)  [unwired: 3 out]
                                n900 = Reciprocal(x=w1939) -> (1/x=w1938:dbl)
                                n901 = Compound Arithmetic op=MULTIPLY(w1936, 255.0 ("value"), w1938) -> (w1934:dbl[])
                                n902 = To Unsigned Byte Integer(number=w1934) -> (unsigned 8bit integer=w1935:u8[])
                                n903 = call "ORS_DrawFlattenedPixmap8.vi"("colormap data string"=w1944, "height"=w1942, "width"=w1941, "image data"=w1935) -> ()  [unwired: 5 in, 1 out]
                                }
                                }
                                }
                                }
                                n904 = local write "new picture"(w1899) -> ()
                                }
                              }
                            }
                            n905 = Unbundle By Name(w1802) -> ("Misc_I/O"=w1787:enum16{"FDML", "NI_DAQ", "None"})
                            n906 = case shown="\"NI_DAQ\"" w1787 {
                              tunnel: TRUE ("data") -> [_ w1804]
                              tunnel: w1802 -> [_ w1803]
                              frame "FDML", Default {
                              }
                              frame "NI_DAQ" {
                                n907 = Unbundle By Name(w1803) -> ("shutter2"=w1806:refnum<k21>)
                                n908 = call-poly <vilib>:"DAQmx Write.vi"("task/channels in"=w1806, "auto start"=TRUE, "data"=w1804) -> ()  [unwired: 10 in, 3 out]
                              }
                            }
                          }
                          frame #2 {
                            n909 = Release Queue(queue=w1947) -> ()  [unwired: 2 in, 3 out]
                          }
                        }
                        n910 = Tick Count (ms)() -> (millisecond timer value=w1698:u32)
                      }
                      frame #3 {
                        # "close file"
                        n911 = local read "Write data?"() -> (w1956:bool)
                        n912 = local read "ATSHandle"() -> (w1951:u32[])
                        n913 = local write "Start 3D scan"(FALSE) -> ()
                        n914 = local write "cancel 3D"(FALSE) -> ()
                        n915 = Subtract(x=w1960, y=w1961) -> (x-y=→"3d acq time":u32)
                        n916 = Subtract(x=w1957, y=w1960) -> (x-y=→"transfer time":u32)
                        n917 = for {
                          tunnel: w1951 -> [w1967] mode=indexing
                          shift-right: [w1968] -> w1954
                          shift-left: w1950 -> [w1965]
                          n918 = call "AlazarAbortCapture.vi"("Handle"=w1967, "error in (no error)"=w1965) -> ("Handle"=w1966:u32, "error out"=w1964:errorcluster)  [unwired: 1 out]
                          n919 = call "AlazarAbortAsyncRead.vi"("Handle"=w1966, "error in (no error)"=w1964) -> ("error out"=w1968:errorcluster)  [unwired: 2 out]
                        }
                        n920 = case shown="True" w1956 {
                          tunnel: w1955 -> [_ w1972]
                          tunnel: w1953 -> [w1969 w1971]
                          tunnel: [w1969 w1970] -> w1952
                          frame False {
                          }
                          frame True {
                            n921 = call "ORS_DatafileClose.vi"("error in"=w1971, "file refnum"=w1972) -> ("error out"=w1970:errorcluster)  [unwired: 9 in]
                          }
                        }
                        n922 = call <vilib>:"Simple Error Handler.vi"("error in (no error)"=w1952) -> ()  [unwired: 4 in, 5 out]
                        n923 = call <vilib>:"Simple Error Handler.vi"("error in (no error)"=w1954) -> ()  [unwired: 4 in, 5 out]
                      }
                      frame #4 {
                        w1986 = FALSE  # open sample arm
                        n924 = local read "scan_flip_state"() -> (w1974:bool)
                        n925 = local write "Apply Config"(TRUE) -> ()
                        n926 = local write "Start 3D scan"(FALSE ("Start 3D scan")) -> ()
                        n927 = Not(x=w1974) -> (.not. x?=w1973:bool)
                        n928 = local write "scan_flip_state"(w1973) -> ()
                        n929 = Unbundle By Name(w1985) -> ("Galvo"=w1983:T5)
                        n930 = local read "XY: Force zero"() -> (w1980:bool)
                        n931 = local read "# lines"() -> (w1982:i32)
                        n932 = call "ORS_GalvoCleanupScan.vi"("Galvo"=w1983) -> ("error out"=w1978:errorcluster, "Galvo out"=w1981:T5)  [unwired: 9 in]
                        n933 = Unbundle By Name(w1985) -> ("Misc_I/O"=w1984:enum16{"FDML", "NI_DAQ", "None"})
                        n934 = call "ORS_GalvoConfig2D_uw.vi"("Galvo"=w1981, "force to zero"=w1980, "n_lines"=w1982, "error in"=w1978) -> ("Galvo out"=w1979:T5)  [unwired: 10 in, 1 out]
                        n935 = case shown="\"NI_DAQ\"" w1984 {
                          tunnel: w1986 -> [_ w1991]
                          tunnel: w1985 -> [_ w1988]
                          frame "FDML", "None", Default {
                          }
                          frame "NI_DAQ" {
                            n936 = Unbundle By Name(w1988) -> ("shutter2"=w1989:refnum<k21>)
                            n937 = call-poly <vilib>:"DAQmx Write.vi"("task/channels in"=w1989, "auto start"=TRUE, "data"=w1991) -> ()  [unwired: 10 in, 3 out]
                          }
                        }
                        n938 = Bundle By Name(cluster=w1985, "Galvo"=w1979) -> (w1987:T6)
                      }
                    }
                  }
                  frame "none", Default {
                    # "This case intentionally does nothing."
                    n939 = local write "Apply Acq Config"(TRUE ("Apply Acq Config")) -> ()
                  }
                }
              }
            }
            n940 = feedback-in #2(w872) -> ()
          }
        }
        n941 = Or(x="exit", y=w90) -> (x .or. y?=w73:bool)
        "Main loop" <- w89
      }
      n942 = feedback-in #1(w56) -> ()
    }
    frame #2 {
      # "system deinit/cleanup"
      n943 = Unbundle By Name(w1997) -> ("shutter1"=w2001:refnum<k21>)
      n944 = Unbundle By Name(w1997) -> ("shutter2"=w2000:refnum<k21>)
      n945 = local write "exit"(FALSE ("exit")) -> ()
      n946 = call <vilib>:"DAQmx Clear Task.vi"("task in"=w2001) -> ()  [unwired: 14 in, 1 out]
      n947 = call <vilib>:"DAQmx Clear Task.vi"("task in"=w2000) -> ()  [unwired: 14 in, 1 out]
      n948 = local read "ATSHandle"() -> (w1995:u32[])
      n949 = Unbundle By Name(w1997) -> ("Galvo"=w1998:T5, "Galvo.FDML-box"=w1996:refnum<visa-resource-name>)
      n950 = call "ORS_GalvoClose.vi"("Galvo"=w1998) -> ()  [unwired: 9 in, 1 out]
      n951 = flat-sequence {
        tunnel: w1996 -> [w2005]
        tunnel: [w2005] -> _
        frame #0 {
          w2003 = T14 0 items=["no dialog", "OK message", "continue or stop message", "OK message + warnings", "continue/stop + warnings"] ("type of dialog (OK msg:1)")
          n952 = VISA Close(VISA resource name=w2005) -> (error out=w2004:errorcluster)  [unwired: 1 in]
          n953 = call <vilib>:"Simple Error Handler.vi"("type of dialog (OK msg:1)"=w2003, "error in (no error)"=w2004) -> ()  [unwired: 3 in, 5 out]
        }
      }
      n954 = for {
        tunnel: w1995 -> [w2002] mode=indexing
        n955 = call "AlazarAbortAsyncRead.vi"("Handle"=w2002) -> ()  [unwired: 1 in, 3 out]
      }
    }
  }
